vi "matlab_TI2_getXYZpos.vi"(8 "error in":errorcluster) -> (0 "error out":errorcluster, 2 "XYZpos":cluster{dbl, dbl, dbl})   [LabVIEW 2018]
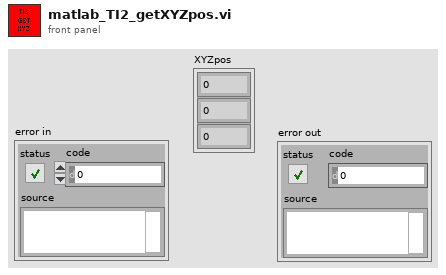
[diagram p1: front panel]
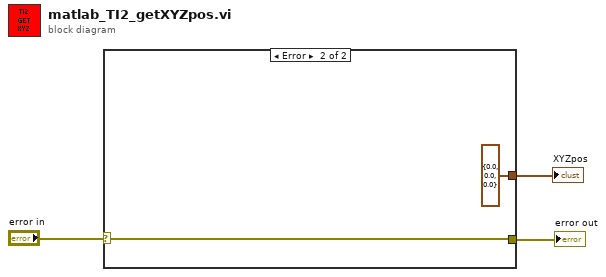
[diagram p0: block diagram]
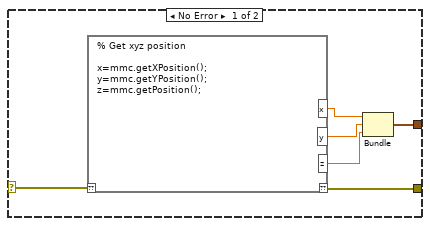
[diagram p2: hidden frame]
diagram:
  n1 = case shown="Error" "error in" {
    selector: "error in" -> [w9 w11]
    tunnel: [w8 w11] -> w2
    tunnel: [w5 cluster{dbl, dbl, dbl} {0.0, 0.0, 0.0}] -> w1
    frame No Error {
      n2 = script code="% Get xyz position\n\nx=mmc.getXPosition();\ny=mmc.getYPosition();\nz=mmc.getPosition();"("??"=w9) -> ("??"=w8:errorcluster, "x"=w7:dbl, "y"=w6:dbl, "z"=w4:dbl)
      n3 = Bundle(w7, w6, w4) -> (w5:cluster{dbl, dbl, dbl})  [unwired: 1 in]
    }
    frame Error {
    }
  }
  "error out" <- w2
  "XYZpos" <- w1
